vi "PH_Cont-601k_PSU.set i Attr and open Services.vi"(0 "i ref in":refnum<vi>, 5 "error in":errorcluster) -> (14 "i ref out":refnum<vi>, 17 "i Attributes":T1={"GUI Refs"={"Power On"=refnum, "Hard- and Software"=refnum, "Device Status"=refnum, "Device Error"=refnum, "Configuration"=refnum, "Flash Interval [s]"=refnum, "Interlock"=refnum, "Interlock Indicator"=refnum, "Voltage [V]"=refnum, "Readyness"=refnum, "Mode"=refnum, "Reset Error"=refnum, "Expert working"=refnum, "Charge"=refnum, "PSU On"=refnum}, "Interlock"=FALSE, "Service ID applied Voltage"=-1, "Device Settings"={"Configuration"=6, "Flash Interval [s]"=30.0, "Mode"=enum."STOP", "Voltage [V]"=0, "Charge"=FALSE, "VISA resource name"="COM1"}, "Readyness"={"Program"=enum."OFF", "Device"=enum."OFF"}, "Information"={"VISA resource name"="COM1", "Tagname Power On"="", "Interlock"={"Instance"="", "Tagname"=""}, "Limits [V]"={"Lower"=0.0, "Upper"=0.0}, "Tagname PSU On"=""}, "R2S"=FALSE, "Charge is allowed"=FALSE} {"Device Settings"."Voltage [V]" max=2000 step=10; "Device Settings"."Flash Interval [s]" min=5.0 max=60.0 step=1.0; "Device Settings"."Configuration" items=["Ch intl, Fl intl, QSw intl", "Ch intl, Fl intl, QSw ext", "Ch intl, Fl ext, QSw intl", "Ch intl, Fl ext, QSw ext", "Ch ext, Fl int, QSw int", "Ch ext, Fl int, QSw ext", "Ch ext, Fl ext, QSw int", "Ch ext, Fl ext, QSw ext"]}, 19 "error out":errorcluster)   [LabVIEW 2014, in "PH_Cont-601k_PSU.lvlib"]
uses:
  PH_Cont-601k_PSU.lvlib
  PH_Cont-601k_PSU.i attribute.ctl
  PH_Cont-601k_PSU.GUI Refs.ctl
  PH_Cont-601k_PSU.Device Status.ctl
  PH_Cont-601k_PSU.Readyness.ctl
  PH_Cont-601k_PSU.Readyness Program.ctl
  PH_Cont-601k_PSU.Readyness Device.ctl
  PH_Cont-601k_PSU.Mode.ctl
  PH_Cont-601k_PSU.Configuration.ctl
  PH_PP_Common/PH_PP_Common.PSU Tags.ctl
  PH_PP_Common/PH_PP_Common.PUs.ctl
  PH_PP_Common/PH_PP_Common.lvlib
  lib.lib/DimLVEvent/LVDimInterface/LVDimInterface.lvlib
  PH_Common/PH_Common.lvlib
  CSCore/CSSystem/CSSystemLib/CSSystemLib.lvlib
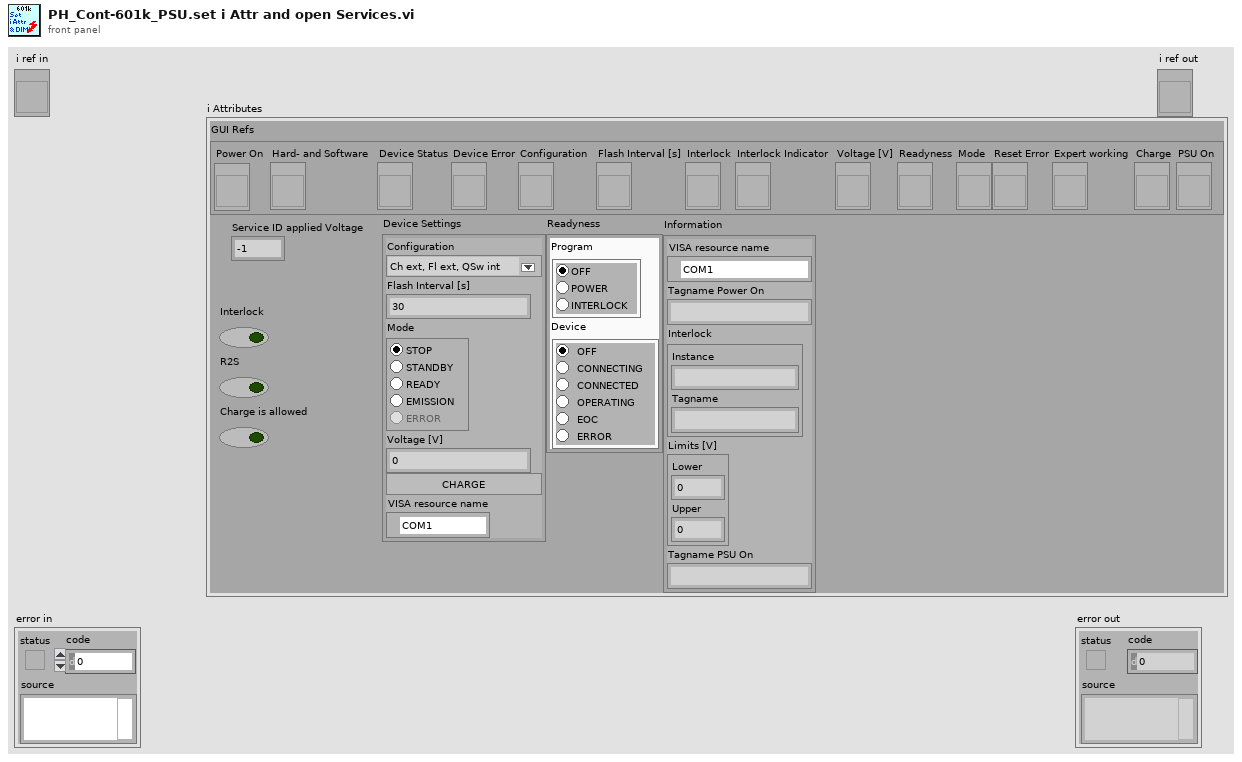
[diagram p1: front panel]
types:
  T1 = typedef "PH_Cont-601k_PSU.lvlib/PH_Cont-601k_PSU.i attribute.ctl" = cluster{"GUI Refs":T2, "Interlock":bool, "Service ID applied Voltage":i32, "Device Settings":cluster{"Configuration":T3, "Flash Interval [s]":dbl, "Mode":T4, "Voltage [V]":u16, "Charge":bool, "VISA resource name":refnum<visa-resource-name>}, "Readyness":T5, "Information":cluster{"VISA resource name":refnum<visa-resource-name>, "Tagname Power On":string, "Interlock":cluster{"Instance":string, "Tagname":string}, "Limits [V]":cluster{"Lower":dbl, "Upper":dbl}, "Tagname PSU On":string}, "R2S":bool, "Charge is allowed":bool}
  T2 = typedef "PH_Cont-601k_PSU.lvlib/PH_Cont-601k_PSU.GUI Refs.ctl" = cluster{"Power On":refnum<vi>, "Hard- and Software":refnum<vi>, "Device Status":refnum<vi>, "Device Error":refnum<vi>, "Configuration":refnum<vi>, "Flash Interval [s]":refnum<vi>, "Interlock":refnum<vi>, "Interlock Indicator":refnum<vi>, "Voltage [V]":refnum<vi>, "Readyness":refnum<vi>, "Mode":refnum<vi>, "Reset Error":refnum<vi>, "Expert working":refnum<vi>, "Charge":refnum<vi>, "PSU On":refnum<vi>}
  T3 = typedef "PH_Cont-601k_PSU.lvlib/PH_Cont-601k_PSU.Configuration.ctl" = u16
  T4 = typedef "PH_Cont-601k_PSU.lvlib/PH_Cont-601k_PSU.Mode.ctl" = enum32{"STOP", "STANDBY", "READY", "EMISSION", "ERROR"}
  T5 = typedef "PH_Cont-601k_PSU.lvlib/PH_Cont-601k_PSU.Readyness.ctl" = cluster{"Program":T6, "Device":T7}
  T6 = typedef "PH_Cont-601k_PSU.lvlib/PH_Cont-601k_PSU.Readyness Program.ctl" = enum32{"OFF", "POWER", "INTERLOCK"}
  T7 = typedef "PH_Cont-601k_PSU.lvlib/PH_Cont-601k_PSU.Readyness Device.ctl" = enum32{"OFF", "CONNECTING", "CONNECTED", "OPERATING", "EOC", "ERROR"}
  T8 = typedef "PH_PP_Common.lvlib/PH_PP_Common.PSU Tags.ctl" = enum16{"voltage-indicator", "peak-detect", "current", "voltage", "inihibit-indicator", "end-of-charge", "HV-on-indicator", "overtemperature", "interlock-indicator", "load-fault", "sum-fault", "HV-off-indicator", "DC-ok", "inhibit", "HV-on", "interlock", "reset", "Status", "Limits"}
  T9 = typedef "PH_PP_Common.lvlib/PH_PP_Common.PUs.ctl" = enum16{"no Info", "PA-19mm-1", "PA-19mm-2", "PA-45mm-PILC", "PA-45mm-MAIN", "MA-PU-1", "MA-PU-2", "MA-PU-3", "MA-PU-4", "MA-PU-5", "MA-PU-6", "MA-FR", "MA-PILC", "PA-45mm-DP"}
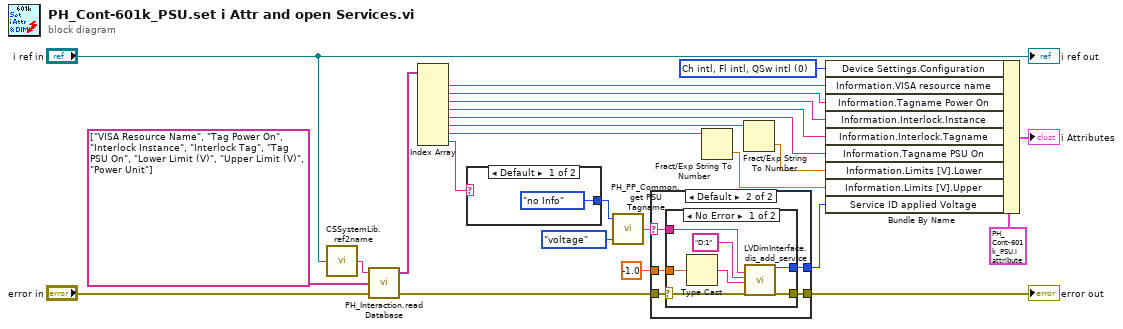
[diagram p0: block diagram]
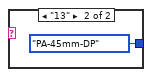
[diagram p2: hidden frame]
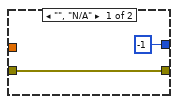
[diagram p3: hidden frame]
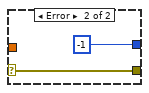
[diagram p4: hidden frame]
diagram:
  w5 = T3 0 items=["Ch intl, Fl intl, QSw intl", "Ch intl, Fl intl, QSw ext", "Ch intl, Fl ext, QSw intl", "Ch intl, Fl ext, QSw ext", "Ch ext, Fl int, QSw int", "Ch ext, Fl int, QSw ext", "Ch ext, Fl ext, QSw int", "Ch ext, Fl ext, QSw ext"] ("Device Settings.Configuration")
  n1 = call "CSSystemLib.ref2name.vi"("obj refnum"="i ref in") -> ("name"=w17:string)
  n2 = call "PH_Interaction.read Database.vi"("error in (no error)"="error in", "Strings to search for"=string[] ["VISA Resource Name", "Tag Power On", "Interlock Instance", "Interlock Tag", "Tag PSU On", "Lower Limit (V)", "Upper Limit (V)", "Power Unit"] ("Strings to search for in"), "DB Entry to read"=w17) -> ("error out"=w7:errorcluster, "Values"=w16:string[])  [unwired: 1 in]
  n3 = Index Array(array=w16) -> (element #1=w15:string, element #2=w14:string, element #3=w13:string, element #4=w12:string, element #5=w1:string, element #6=w2:string, element #7=w3:string, element #8=w4:string)  [unwired: 8 in]
  n4 = case shown="Default" w4 {
    tunnel: [PH_PP_Common.PUs."no Info" ("PU") PH_PP_Common.PUs."PA-45mm-DP" ("PU")] -> w9
    frame Default {
    }
    frame "13" {
    }
  }
  n5 = call "PH_PP_Common.get PSU Tagname.vi"("PSU Tag"=PH_PP_Common.PSU_Tags."voltage", "PU"=w9) -> ("PSU Tagname"=w22:string)  [unwired: 1 in]
  n6 = case shown="Default" w22 {
    selector: w22 -> [_ w30]
    tunnel: [-1 ("my_serviceID") w34] -> w20
    tunnel: -1.0 ("number") -> [_ w33]
    tunnel: w7 -> [w28 w32]
    tunnel: [w28 w31] -> w21
    frame "", "N/A" {
    }
    frame Default {
      n7 = case shown="No Error" w32 {
        selector: w32 -> [w40 w43]
        tunnel: [w36 -1 ("my_serviceID")] -> w34
        tunnel: [w41 w43] -> w31
        tunnel: w33 -> [w35 _]
        tunnel: w30 -> [w38 _]
        frame No Error {
          n8 = Type Cast(x=w35) -> (*(type *) &x=w37:string)  [unwired: 1 in]
          n9 = call "LVDimInterface.dis_add_service.vi"("serviceName"=w38, "typeDescriptor"="D:1", "data"=w37, "error in (no error)"=w40) -> ("my_serviceID"=w36:i32, "error out"=w41:errorcluster)  [unwired: 14 in]
        }
        frame Error {
        }
      }
    }
  }
  "error out" <- w21
  n10 = Fract/Exp String To Number(string=w3) -> (number=w10:dbl)  [unwired: 3 in, 1 out]
  n11 = Fract/Exp String To Number(string=w2) -> (number=w11:dbl)  [unwired: 3 in, 1 out]
  n12 = Bundle By Name(cluster=T1 {"GUI Refs"={"Power On"=refnum, "Hard- and Software"=refnum, "Device Status"=refnum, "Device Error"=refnum, "Configuration"=refnum, "Flash Interval [s]"=refnum, "Interlock"=refnum, "Interlock Indicator"=refnum, "Voltage [V]"=refnum, "Readyness"=refnum, "Mode"=refnum, "Reset Error"=refnum, "Expert working"=refnum, "Charge"=refnum, "PSU On"=refnum}, "Interlock"=FALSE, "Service ID applied Voltage"=-1, "Device Settings"={"Configuration"=6, "Flash Interval [s]"=30.0, "Mode"=enum."STOP", "Voltage [V]"=0, "Charge"=FALSE, "VISA resource name"="COM1"}, "Readyness"={"Program"=enum."OFF", "Device"=enum."OFF"}, "Information"={"VISA resource name"="COM1", "Tagname Power On"="", "Interlock"={"Instance"="", "Tagname"=""}, "Limits [V]"={"Lower"=0.0, "Upper"=0.0}, "Tagname PSU On"=""}, "R2S"=FALSE, "Charge is allowed"=FALSE} ("i attribute"), "Device Settings.Configuration"=w5, "Information.VISA resource name"=w15, "Information.Tagname Power On"=w14, "Information.Interlock.Instance"=w13, "Information.Interlock.Tagname"=w12, "Information.Tagname PSU On"=w1, "Information.Limits [V].Lower"=w11, "Information.Limits [V].Upper"=w10, "Service ID applied Voltage"=w20) -> (→"i Attributes":T1)
  "i ref out" <- "i ref in"
